vi "Generate FilenameUS.vi"(8 "error in":errorcluster, 11 "Log in":refnum<class "Log.lvclass">) -> (0 "error out":errorcluster, 3 "Log out":refnum<class "Log.lvclass">)   [LabVIEW 2017, in "Reports.lvlib" / "Log.lvclass"]
doc: "This SubVI generate filename based on\ncurrent data by polimorphic GenFilename.vi"
uses:
  Log.lvclass
  Log.lvclass/Log.ctl
  <vilib>/regexp/Match Regular Expression.xnode
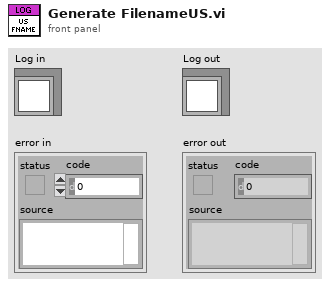
[diagram p1: front panel]
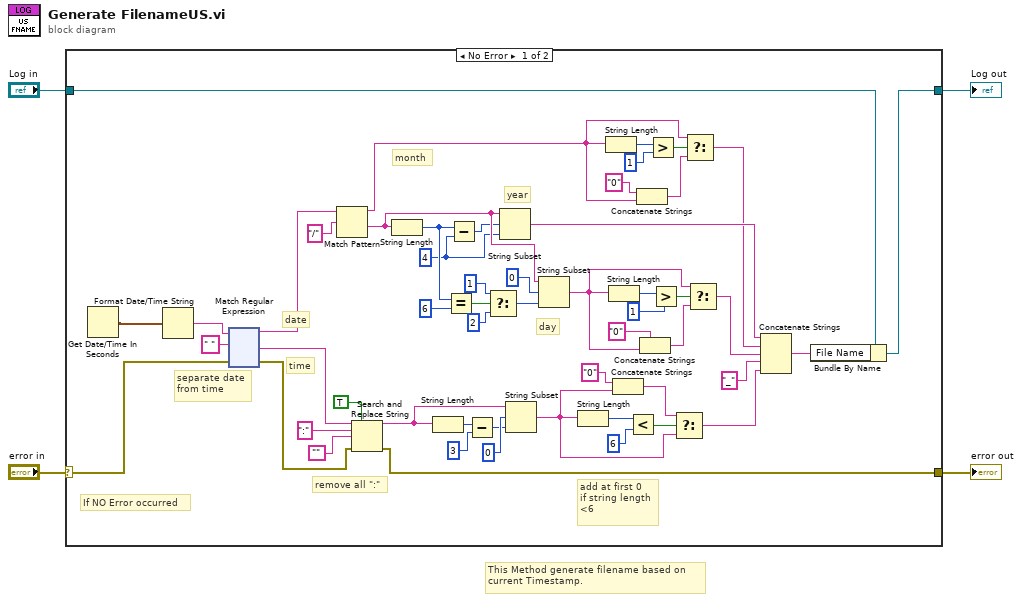
[diagram p0: block diagram]
diagram:
  # "This Method generate filename based on\ncurrent Timestamp."
  n1 = case shown="No Error" "error in" {
    selector: "error in" -> [w54 w173]
    tunnel: [w52 w173] -> w3
    tunnel: [w56 w172] -> w1
    tunnel: "Log in" -> [w57 w172]
    frame No Error {
      w23 = 4 ("y")
      # "day"
      # "month"
      # "year"
      # "add at first 0\nif string length\n<6"
      # "remove all \":\""
      # "separate date \nfrom time"
      # "time"
      # "date"
      # "If NO Error occurred"
      n2 = Get Date/Time In Seconds() -> (seconds since 1Jan1904=w55:timestamp)
      n3 = Format Date/Time String(seconds (now)=w55) -> (date/time string=w51:string)  [unwired: 2 in]
      n4 = xnode "Match Regular Expression"("input string"=w51, "regular expression"=" ", "error in"=w54) -> ("before match"=w20:string, "after match"=w42:string, "error out"=w39:errorcluster)  [unwired: 3 in, 2 out]
      n5 = Match Pattern(string=w20, regular expression="/") -> (before substring=w6:string, after substring=w31:string)  [unwired: 1 in, 2 out]
      n6 = Search and Replace String(replace all?=TRUE ("replace all? (F)"), input string=w42, search string=":", replace string="", error in=w39) -> (result string=w33:string, error out=w52:errorcluster)  [unwired: 3 in, 2 out]
      n7 = String Length(string=w31) -> (length=w24:i32)
      n8 = String Length(string=w33) -> (length=w34:i32)
      n9 = Equal?(x=w24, y=6) -> (x = y?=w26:bool)
      n10 = Subtract(x=w24, y=w23) -> (x-y=w22:i32)
      n11 = Subtract(x=w34, y=3) -> (x-y=w36:i32)
      n12 = Select(t=1 ("y"), s=w26, f=2 ("y")) -> (s? t:f=w29:i32)
      n13 = String Subset(string=w31, offset (0)=w22, length (rest)=w23) -> (substring=w19:string)
      n14 = String Subset(string=w33, offset (0)=0, length (rest)=w36) -> (substring=w32:string)
      n15 = String Subset(string=w31, offset (0)=0, length (rest)=w29) -> (substring=w13:string)
      n16 = String Length(string=w32) -> (length=w44:i32)
      n17 = String Length(string=w6) -> (length=w11:i32)
      n18 = String Length(string=w13) -> (length=w16:i32)
      n19 = Concatenate Strings("0" ("string"), w32) -> (w48:string)
      n20 = Less?(x=w44, y=6) -> (x < y?=w46:bool)
      n21 = Concatenate Strings("0" ("string"), w6) -> (w9:string)
      n22 = Concatenate Strings("0" ("string"), w13) -> (w18:string)
      n23 = Greater?(x=w11, y=1) -> (0:w10:bool)
      n24 = Greater?(x=w16, y=1) -> (0:w17:bool)
      n25 = Select(t=w48, s=w46, f=w32) -> (s? t:f=w50:string)
      n26 = Select(t=w6, s=w10, f=w9) -> (s? t:f=w5:string)
      n27 = Select(t=w13, s=w17, f=w18) -> (s? t:f=w12:string)
      n28 = Concatenate Strings(w19, w5, w12, "_" ("string"), w50) -> (w53:string)
      n29 = Bundle By Name(cluster=w57, "File Name"=w53) -> (w56:refnum<class "Log.lvclass">)
    }
    frame Error {
    }
  }
  "error out" <- w3
  "Log out" <- w1
